vi "FYP_VI_MIDI_Virtual_Piano.vi"() -> ()   [LabVIEW 2013]
doc: "Virtual piano with LabView \nVirtual piano Demo\nMIDI\n\nUse at your own Risk"
uses:
  <vilib>/Utility/file.llb/Write To Spreadsheet File (string).vi
panel:
  in  "Exit":bool
  in  "Export File":bool
  in  "Time":u32
  in  "Table":string[][](table)
  in  "Instrument":i32(listbox)
  in  "Velocity / Volume":u32=127 max=127
  in  "MIDI Channel":u32=1 min=1 max=16
  in  "deviceID":u32
  out "MIDI Note Number":i16
  out "ScanCode":i16
  out ";":bool
  out "L":bool
  out "J":bool
  out "H":bool
  out "G":bool
  out "D":bool
  out "RShift":bool
  out "/":bool
  out ".":bool
  out ",":bool
  out "M":bool
  out "N":bool
  out "B":bool
  out "V":bool
  out "C":bool
  out "Back/S":bool
  out "X":bool
  out "-/CAP":bool
  out "0":bool
  out "9":bool
  out "7":bool
  out "6":bool
  out "4":bool
  out "3":bool
  out "2":bool
  out "]/Z":bool
  out "[/Shift":bool
  out "P":bool
  out "O":bool
  out "I":bool
  out "U":bool
  out "Y":bool
  out "T":bool
  out "R":bool
  out "E":bool
  out "W":bool
  out "Q":bool
  out "~":bool
  out "Tab":bool
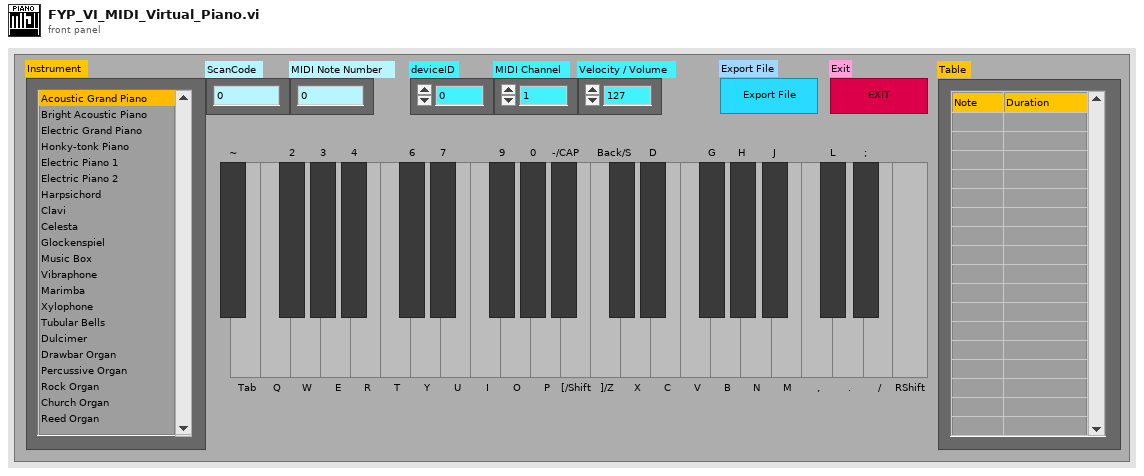
[diagram p1: front panel]
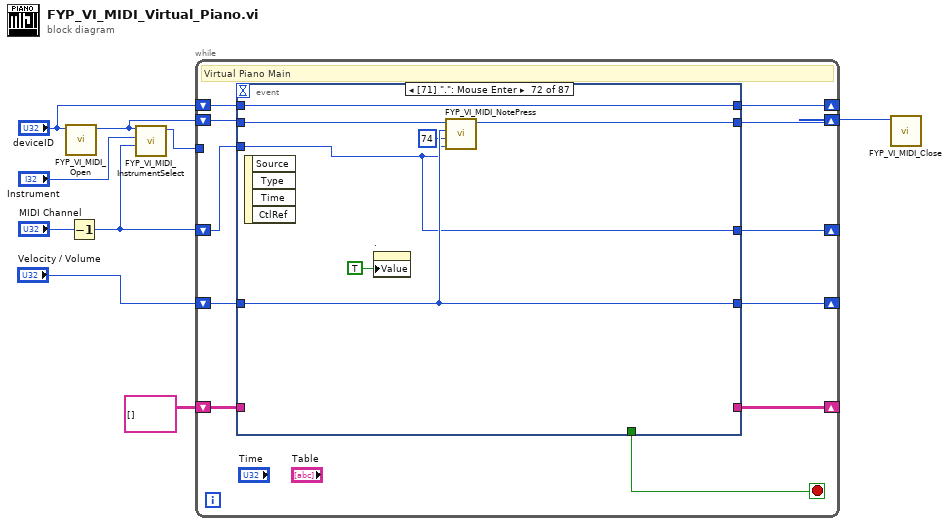
[diagram p0: block diagram]
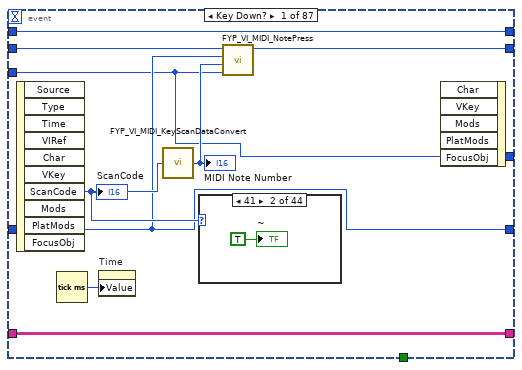
[diagram p2: hidden frame]
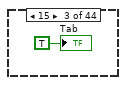
[diagram p4: hidden frame]
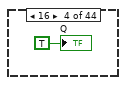
[diagram p5: hidden frame]
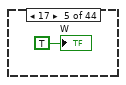
[diagram p6: hidden frame]
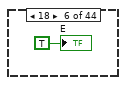
[diagram p7: hidden frame]
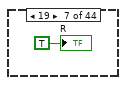
[diagram p8: hidden frame]
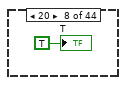
[diagram p9: hidden frame]
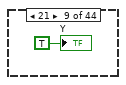
[diagram p10: hidden frame]
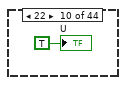
[diagram p11: hidden frame]
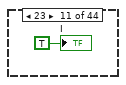
[diagram p12: hidden frame]
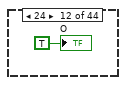
[diagram p13: hidden frame]
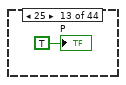
[diagram p14: hidden frame]
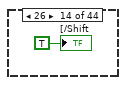
[diagram p15: hidden frame]
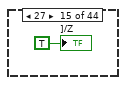
[diagram p16: hidden frame]
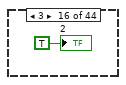
[diagram p17: hidden frame]
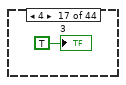
[diagram p18: hidden frame]
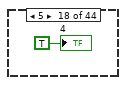
[diagram p19: hidden frame]
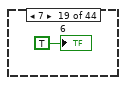
[diagram p20: hidden frame]
diagram:
  n1 = call "FYP_VI_MIDI_Open.vi"("deviceID"="deviceID") -> ("midiOut"=w5:i32)  [unwired: 5 in, 1 out]
  n2 = Decrement(x="MIDI Channel") -> (x-1=w1:u32)
  n3 = call "FYP_VI_MIDI_InstrumentSelect.vi"("MIDI Channel"=w1, "Instrument"="Instrument", "midiOut handle"=w5) -> ("midiOut handle"=w6:i32)  [unwired: 3 in, 1 out]
  n4 = while {
    shift-right: [w19] -> w8
    shift-left: w5 -> [w20]
    shift-right: [w17] -> _
    shift-left: "Velocity / Volume" -> [w18]
    tunnel: w6 -> [_]
    shift-right: [w13] -> _
    shift-left: string[][] [] ("array") -> [w14]
    shift-right: [w11] -> _
    shift-left: "deviceID" -> [w12]
    shift-right: [w10] -> _
    shift-left: w1 -> [w16]
    stop <- w15 stop-if-true
    # "Virtual Piano Main"
    n5 = event shown="[71] \".\": Mouse Enter" {
      selector: _ -> [_ _ _ _ _ _ _ _ _ _ _ _ _ _ _ _ _ _ _ _ _ _ _ _ _ _ _ _ _ _ _ _ _ _ _ _ _ _ _ _ _ _ _ _ _ _ _ _ _ _ _ _ _ _ _ _ _ _ _ _ _ _ _ _ _ _ _ _ _ _ _ _ _ _ _ _ _ _ _ _ _ _ _ _ _ _ _]
      dyn-events: _ -> [_ _ _ _ _ _ _ _ _ _ _ _ _ _ _ _ _ _ _ _ _ _ _ _ _ _ _ _ _ _ _ _ _ _ _ _ _ _ _ _ _ _ _ _ _ _ _ _ _ _ _ _ _ _ _ _ _ _ _ _ _ _ _ _ _ _ _ _ _ _ _ _ _ _ _ _ _ _ _ _ _ _ _ _ _ _ _]
      timeout: _ -> [_ _ _ _ _ _ _ _ _ _ _ _ _ _ _ _ _ _ _ _ _ _ _ _ _ _ _ _ _ _ _ _ _ _ _ _ _ _ _ _ _ _ _ _ _ _ _ _ _ _ _ _ _ _ _ _ _ _ _ _ _ _ _ _ _ _ _ _ _ _ _ _ _ _ _ _ _ _ _ _ _ _ _ _ _ _ _]
      tunnel: w20 -> [w28 w78 w85 w93 w100 w107 w114 w121 w128 w135 w142 w149 w156 w163 w170 w177 w184 w191 w198 w205 w212 w219 w226 w233 w240 w247 w254 w261 w268 w275 w282 w289 w296 w303 w309 w317 w324 w331 w338 w345 w351 w359 w366 w373 w380 w387 w393 w401 w407 w415 w422 w429 w435 w442 w450 w457 w463 w471 w478 w485 w492 w499 w505 w513 w519 w527 w533 w541 w548 w555 w562 w569 w576 w583 w590 w597 w604 w611 w618 w623 w626 w641 w687 w691 w696 w704 w705]
      tunnel: [w27 w77 w84 w92 w99 w106 w113 w120 w127 w134 w141 w148 w155 w162 w169 w176 w183 w190 w197 w204 w211 w218 w225 w232 w239 w246 w253 w260 w267 w274 w281 w288 w295 w302 w308 w316 w323 w330 w337 w344 w350 w358 w365 w372 w379 w386 w392 w400 w406 w414 w421 w428 w434 w441 w449 w456 w462 w470 w477 w484 w491 w498 w500 w512 w518 w526 w532 w540 w547 w554 w561 w563 w575 w582 w589 w596 w603 w610 w617 w623 w626 w640 w689 w691 w696 w703 w705] -> w19
      tunnel: w18 -> [w26 w76 w83 w90 w98 w105 w112 w119 w126 w133 w140 w147 w154 w161 w168 w174 w182 w189 w196 w203 w210 w217 w224 w231 w238 w245 w251 w259 w266 w273 w280 w287 w294 w301 w307 w315 w322 w329 w336 w342 w349 w357 w364 w371 w378 w385 w391 w399 w405 w413 w420 w427 w433 w440 w448 w455 w461 w469 w475 w483 w490 w497 w504 w510 w517 w525 w531 w539 w546 w553 w560 w568 w574 w581 w588 w595 w602 w609 w616 w622 w627 w639 w688 _ w698 w700 w708]
      tunnel: [w26 w76 w83 w90 w98 w105 w112 w119 w126 w133 w140 w147 w154 w161 w168 w174 w182 w189 w196 w203 w210 w217 w224 w231 w238 w245 w251 w259 w266 w273 w280 w287 w294 w301 w307 w315 w322 w329 w336 w342 w349 w357 w364 w371 w378 w385 w391 w399 w405 w413 w420 w427 w433 w440 w448 w455 w461 w469 w475 w483 w490 w497 w504 w510 w517 w525 w531 w539 w546 w553 w560 w568 w574 w581 w588 w595 w602 w609 w616 w622 w627 w639 w688 w694 w698 w700 w708] -> w17
      tunnel: w16 -> [w21 w74 w81 w87 w95 w101 w108 w115 w122 w129 w136 w143 w150 w157 w164 w171 w178 w186 w192 w200 w206 w213 w220 w227 w234 w241 w248 w255 w262 w269 w276 w283 w290 w297 w305 w312 w319 w326 w332 w339 w346 w353 w361 w367 w374 w381 w388 w395 w402 w409 w416 w423 w430 w437 w444 w451 w458 w465 w472 w480 w487 w493 w501 w507 w514 w521 w528 w535 w542 w549 w556 w564 w570 w577 w584 w591 w599 w605 w612 w621 w625 w629 w686 w693 _ w701 w707]
      tunnel: [_ _ _ _ _ _ _ _ _ _ _ _ _ _ _ _ _ _ _ _ _ _ _ _ _ _ _ _ _ _ _ _ _ _ _ _ _ _ _ _ _ _ _ _ _ _ _ _ _ _ _ _ _ _ _ _ _ _ _ _ _ _ _ _ _ _ _ _ _ _ _ _ _ _ _ _ _ _ _ "Exit" _ _ _ _ _ _ _] -> w15
      tunnel: w14 -> [w23 _ _ _ _ _ _ _ _ _ _ _ _ _ _ _ _ _ _ _ _ _ _ _ _ _ _ _ _ _ _ _ _ _ _ _ _ _ _ _ _ _ _ _ _ _ _ _ _ _ _ _ _ _ _ _ _ _ _ _ _ _ _ _ _ _ _ _ _ _ _ _ _ _ _ _ _ _ _ _ _ w634 _ _ _ _ w713]
      tunnel: [w23 _ _ _ _ _ _ _ _ _ _ _ _ _ _ _ _ _ _ _ _ _ _ _ _ _ _ _ _ _ _ _ _ _ _ _ _ _ _ _ _ _ _ _ _ _ _ _ _ _ _ _ _ _ _ _ _ _ _ _ _ _ _ _ _ _ _ _ _ _ _ _ _ _ _ _ _ _ _ _ _ w631 _ _ _ _ _] -> w13
      tunnel: w12 -> [w22 w73 w80 w88 w94 w102 w109 w116 w123 w130 w137 w144 w151 w158 w165 w172 w179 w185 w193 w199 w207 w214 w221 w228 w235 w242 w249 w256 w263 w270 w277 w284 w291 w298 w304 w311 w318 w325 w333 w340 w347 w354 w360 w368 w375 w382 w389 w396 w403 w410 w417 w424 w431 w438 w445 w452 w459 w466 w473 w479 w486 w494 w502 w508 w515 w522 w529 w536 w543 w550 w557 w565 w571 w578 w585 w592 w598 w606 w613 w620 w624 w630 w685 w692 w697 w702 w706]
      tunnel: [w22 w73 w80 w88 w94 w102 w109 w116 w123 w130 w137 w144 w151 w158 w165 w172 w179 w185 w193 w199 w207 w214 w221 w228 w235 w242 w249 w256 w263 w270 w277 w284 w291 w298 w304 w311 w318 w325 w333 w340 w347 w354 w360 w368 w375 w382 w389 w396 w403 w410 w417 w424 w431 w438 w445 w452 w459 w466 w473 w479 w486 w494 w502 w508 w515 w522 w529 w536 w543 w550 w557 w565 w571 w578 w585 w592 w598 w606 w613 w620 w624 w630 w685 w692 w697 w702 w706] -> w11
      tunnel: [w21 w74 w81 w87 w95 w101 w108 w115 w122 w129 w136 w143 w150 w157 w164 w171 w178 w186 w192 w200 w206 w213 w220 w227 w234 w241 w248 w255 w262 w269 w276 w283 w290 w297 w305 w312 w319 w326 w332 w339 w346 w353 w361 w367 w374 w381 w388 w395 w402 w409 w416 w423 w430 w437 w444 w451 w458 w465 w472 w480 w487 w493 w501 w507 w514 w521 w528 w535 w542 w549 w556 w564 w570 w577 w584 w591 w599 w605 w612 w621 w625 w629 w686 w693 w695 w701 w707] -> w10
      event Key Down? {
        n6 = event-data() -> ("ScanCode"=w29:i16)  [unwired: 1 in, 9 out]
        "ScanCode" <- w29
        n7 = Tick Count (ms)() -> (millisecond timer value=w24:u32)
        n8 = property on="Time" class="DigNum (strict)"("Value"=w24) -> ()  [unwired: 2 in, 2 out]
        n9 = call "FYP_VI_MIDI_KeyScanDataConvert.vi"("KeyScan"=w29) -> ("MIDI Note Number"=w25:i16)
        "MIDI Note Number" <- w25
        n10 = case shown="41" w29 {
          frame 0, Default {
          }
          frame 41 {
            "~" <- TRUE ("Q")
          }
          frame 15 {
            "Tab" <- TRUE ("Q")
          }
          frame 16 {
            "Q" <- TRUE ("Q")
          }
          frame 17 {
            "W" <- TRUE ("4")
          }
          frame 18 {
            "E" <- TRUE ("4")
          }
          frame 19 {
            "R" <- TRUE ("4")
          }
          frame 20 {
            "T" <- TRUE ("4")
          }
          frame 21 {
            "Y" <- TRUE ("4")
          }
          frame 22 {
            "U" <- TRUE ("4")
          }
          frame 23 {
            "I" <- TRUE ("4")
          }
          frame 24 {
            "O" <- TRUE ("4")
          }
          frame 25 {
            "P" <- TRUE ("4")
          }
          frame 26 {
            "[/Shift" <- TRUE ("4")
          }
          frame 27 {
            "]/Z" <- TRUE ("4")
          }
          frame 3 {
            "2" <- TRUE ("Q")
          }
          frame 4 {
            "3" <- TRUE ("4")
          }
          frame 5 {
            "4" <- TRUE ("4")
          }
          frame 7 {
            "6" <- TRUE ("4")
          }
          frame 8 {
            "7" <- TRUE ("4")
          }
          frame 10 {
            "9" <- TRUE ("4")
          }
          frame 11 {
            "0" <- TRUE ("4")
          }
          frame 12 {
            "-/CAP" <- TRUE ("4")
          }
          frame 14 {
            "Back/S" <- TRUE ("4")
          }
          frame 58 {
            n11 = property on="-/CAP" class="Bool"("Value"=TRUE ("4")) -> ()  [unwired: 2 in, 2 out]
          }
          frame 42 {
            n12 = local write "[/Shift"(TRUE ("4")) -> ()
          }
          frame 44 {
            n13 = local write "]/Z"(TRUE ("4")) -> ()
          }
          frame 45 {
            "X" <- TRUE ("4")
          }
          frame 46 {
            "C" <- TRUE ("4")
          }
          frame 47 {
            "V" <- TRUE ("4")
          }
          frame 48 {
            "B" <- TRUE ("4")
          }
          frame 49 {
            "N" <- TRUE ("4")
          }
          frame 50 {
            "M" <- TRUE ("4")
          }
          frame 51 {
            "," <- TRUE ("4")
          }
          frame 52 {
            "." <- TRUE ("4")
          }
          frame 53 {
            "/" <- TRUE ("4")
          }
          frame 54 {
            "RShift" <- TRUE ("4")
          }
          frame 31 {
            n14 = local write "Back/S"(TRUE ("4")) -> ()
          }
          frame 32 {
            "D" <- TRUE ("4")
          }
          frame 34 {
            "G" <- TRUE ("4")
          }
          frame 35 {
            "H" <- TRUE ("4")
          }
          frame 36 {
            "J" <- TRUE ("4")
          }
          frame 38 {
            "L" <- TRUE ("4")
          }
          frame 39 {
            ";" <- TRUE ("4")
          }
        }
        n15 = call "FYP_VI_MIDI_NotePress.vi"("MIDI Channel"=w21, "Pitch Note"=w25, "Velocity / Volume"=w26, "midiOut Handle"=w28) -> ("midiOut handle"=w27:i32)  [unwired: 2 in, 1 out]
        n16 = event-data() -> ()  [unwired: 6 in, 1 out]
      }
      event "~": Mouse Enter {
        n17 = event-data() -> ()  [unwired: 1 in, 4 out]
        n18 = property on="~" class="Bool"("Value"=TRUE ("Q")) -> ()  [unwired: 2 in, 2 out]
        n19 = call "FYP_VI_MIDI_NotePress.vi"("MIDI Channel"=w74, "Pitch Note"=u32 39, "Velocity / Volume"=w76, "midiOut Handle"=w78) -> ("midiOut handle"=w77:i32)  [unwired: 2 in, 1 out]
      }
      event "~": Mouse Leave {
        n20 = event-data() -> ()  [unwired: 1 in, 4 out]
        n21 = property on="~" class="Bool"("Value"=FALSE ("Q")) -> ()  [unwired: 2 in, 2 out]
        n22 = call "FYP_VI_MIDI_NoteRelease.vi"("MIDI Channel"=w81, "Pitch Note"=u32 39, "Velocity / Volume"=w83, "midiOut Handle"=w85) -> ("midiOut handle"=w84:i32)  [unwired: 2 in, 1 out]
      }
      event "Tab": Mouse Enter {
        n23 = event-data() -> ()  [unwired: 1 in, 4 out]
        n24 = property on="Tab" class="Bool"("Value"=TRUE ("Q")) -> ()  [unwired: 2 in, 2 out]
        n25 = call "FYP_VI_MIDI_NotePress.vi"("MIDI Channel"=w87, "Pitch Note"=u32 40, "Velocity / Volume"=w90, "midiOut Handle"=w93) -> ("midiOut handle"=w92:i32)  [unwired: 2 in, 1 out]
      }
      event "Tab": Mouse Leave {
        n26 = event-data() -> ()  [unwired: 1 in, 4 out]
        n27 = property on="Tab" class="Bool"("Value"=FALSE ("Q")) -> ()  [unwired: 2 in, 2 out]
        n28 = call "FYP_VI_MIDI_NoteRelease.vi"("MIDI Channel"=w95, "Pitch Note"=u32 40, "Velocity / Volume"=w98, "midiOut Handle"=w100) -> ("midiOut handle"=w99:i32)  [unwired: 2 in, 1 out]
      }
      event "Q": Mouse Enter {
        n29 = event-data() -> ()  [unwired: 1 in, 4 out]
        n30 = property on="Q" class="Bool"("Value"=TRUE ("Q")) -> ()  [unwired: 2 in, 2 out]
        n31 = call "FYP_VI_MIDI_NotePress.vi"("MIDI Channel"=w101, "Pitch Note"=u32 41, "Velocity / Volume"=w105, "midiOut Handle"=w107) -> ("midiOut handle"=w106:i32)  [unwired: 2 in, 1 out]
      }
      event "Q": Mouse Leave {
        n32 = event-data() -> ()  [unwired: 1 in, 4 out]
        n33 = property on="Q" class="Bool"("Value"=FALSE ("Q")) -> ()  [unwired: 2 in, 2 out]
        n34 = call "FYP_VI_MIDI_NoteRelease.vi"("MIDI Channel"=w108, "Pitch Note"=u32 41, "Velocity / Volume"=w112, "midiOut Handle"=w114) -> ("midiOut handle"=w113:i32)  [unwired: 2 in, 1 out]
      }
      event "2": Mouse Enter {
        n35 = event-data() -> ()  [unwired: 1 in, 4 out]
        n36 = property on="2" class="Bool"("Value"=TRUE ("Q")) -> ()  [unwired: 2 in, 2 out]
        n37 = call "FYP_VI_MIDI_NotePress.vi"("MIDI Channel"=w115, "Pitch Note"=u32 42, "Velocity / Volume"=w119, "midiOut Handle"=w121) -> ("midiOut handle"=w120:i32)  [unwired: 2 in, 1 out]
      }
      event "2": Mouse Leave {
        n38 = event-data() -> ()  [unwired: 1 in, 4 out]
        n39 = property on="2" class="Bool"("Value"=FALSE ("Q")) -> ()  [unwired: 2 in, 2 out]
        n40 = call "FYP_VI_MIDI_NoteRelease.vi"("MIDI Channel"=w122, "Pitch Note"=u32 42, "Velocity / Volume"=w126, "midiOut Handle"=w128) -> ("midiOut handle"=w127:i32)  [unwired: 2 in, 1 out]
      }
      event "W": Mouse Enter {
        n41 = event-data() -> ()  [unwired: 1 in, 4 out]
        n42 = property on="W" class="Bool"("Value"=TRUE ("Q")) -> ()  [unwired: 2 in, 2 out]
        n43 = call "FYP_VI_MIDI_NotePress.vi"("MIDI Channel"=w129, "Pitch Note"=u32 43, "Velocity / Volume"=w133, "midiOut Handle"=w135) -> ("midiOut handle"=w134:i32)  [unwired: 2 in, 1 out]
      }
      event "W": Mouse Leave {
        n44 = event-data() -> ()  [unwired: 1 in, 4 out]
        n45 = property on="W" class="Bool"("Value"=FALSE ("Q")) -> ()  [unwired: 2 in, 2 out]
        n46 = call "FYP_VI_MIDI_NoteRelease.vi"("MIDI Channel"=w136, "Pitch Note"=u32 43, "Velocity / Volume"=w140, "midiOut Handle"=w142) -> ("midiOut handle"=w141:i32)  [unwired: 2 in, 1 out]
      }
      event "3": Mouse Enter {
        n47 = event-data() -> ()  [unwired: 1 in, 4 out]
        n48 = property on="3" class="Bool"("Value"=TRUE ("Q")) -> ()  [unwired: 2 in, 2 out]
        n49 = call "FYP_VI_MIDI_NotePress.vi"("MIDI Channel"=w143, "Pitch Note"=u32 44, "Velocity / Volume"=w147, "midiOut Handle"=w149) -> ("midiOut handle"=w148:i32)  [unwired: 2 in, 1 out]
      }
      event "3": Mouse Leave {
        n50 = event-data() -> ()  [unwired: 1 in, 4 out]
        n51 = property on="3" class="Bool"("Value"=FALSE ("Q")) -> ()  [unwired: 2 in, 2 out]
        n52 = call "FYP_VI_MIDI_NoteRelease.vi"("MIDI Channel"=w150, "Pitch Note"=u32 44, "Velocity / Volume"=w154, "midiOut Handle"=w156) -> ("midiOut handle"=w155:i32)  [unwired: 2 in, 1 out]
      }
      event "E": Mouse Enter {
        n53 = event-data() -> ()  [unwired: 1 in, 4 out]
        n54 = property on="E" class="Bool"("Value"=TRUE ("Q")) -> ()  [unwired: 2 in, 2 out]
        n55 = call "FYP_VI_MIDI_NotePress.vi"("MIDI Channel"=w157, "Pitch Note"=u32 45, "Velocity / Volume"=w161, "midiOut Handle"=w163) -> ("midiOut handle"=w162:i32)  [unwired: 2 in, 1 out]
      }
      event "E": Mouse Leave {
        n56 = event-data() -> ()  [unwired: 1 in, 4 out]
        n57 = property on="E" class="Bool"("Value"=FALSE ("Q")) -> ()  [unwired: 2 in, 2 out]
        n58 = call "FYP_VI_MIDI_NoteRelease.vi"("MIDI Channel"=w164, "Pitch Note"=u32 45, "Velocity / Volume"=w168, "midiOut Handle"=w170) -> ("midiOut handle"=w169:i32)  [unwired: 2 in, 1 out]
      }
      event "4": Mouse Enter {
        n59 = event-data() -> ()  [unwired: 1 in, 4 out]
        n60 = property on="4" class="Bool"("Value"=TRUE ("Q")) -> ()  [unwired: 2 in, 2 out]
        n61 = call "FYP_VI_MIDI_NotePress.vi"("MIDI Channel"=w171, "Pitch Note"=u32 46, "Velocity / Volume"=w174, "midiOut Handle"=w177) -> ("midiOut handle"=w176:i32)  [unwired: 2 in, 1 out]
      }
      event "4": Mouse Leave {
        n62 = event-data() -> ()  [unwired: 1 in, 4 out]
        n63 = property on="4" class="Bool"("Value"=FALSE ("Q")) -> ()  [unwired: 2 in, 2 out]
        n64 = call "FYP_VI_MIDI_NoteRelease.vi"("MIDI Channel"=w178, "Pitch Note"=u32 46, "Velocity / Volume"=w182, "midiOut Handle"=w184) -> ("midiOut handle"=w183:i32)  [unwired: 2 in, 1 out]
      }
      event "R": Mouse Enter {
        n65 = event-data() -> ()  [unwired: 1 in, 4 out]
        n66 = property on="R" class="Bool"("Value"=TRUE ("Q")) -> ()  [unwired: 2 in, 2 out]
        n67 = call "FYP_VI_MIDI_NotePress.vi"("MIDI Channel"=w186, "Pitch Note"=u32 47, "Velocity / Volume"=w189, "midiOut Handle"=w191) -> ("midiOut handle"=w190:i32)  [unwired: 2 in, 1 out]
      }
      event "R": Mouse Leave {
        n68 = event-data() -> ()  [unwired: 1 in, 4 out]
        n69 = property on="R" class="Bool"("Value"=FALSE ("Q")) -> ()  [unwired: 2 in, 2 out]
        n70 = call "FYP_VI_MIDI_NoteRelease.vi"("MIDI Channel"=w192, "Pitch Note"=u32 47, "Velocity / Volume"=w196, "midiOut Handle"=w198) -> ("midiOut handle"=w197:i32)  [unwired: 2 in, 1 out]
      }
      event "T": Mouse Enter {
        n71 = event-data() -> ()  [unwired: 1 in, 4 out]
        n72 = property on="T" class="Bool"("Value"=TRUE ("Q")) -> ()  [unwired: 2 in, 2 out]
        n73 = call "FYP_VI_MIDI_NotePress.vi"("MIDI Channel"=w200, "Pitch Note"=u32 48, "Velocity / Volume"=w203, "midiOut Handle"=w205) -> ("midiOut handle"=w204:i32)  [unwired: 2 in, 1 out]
      }
      event "T": Mouse Leave {
        n74 = event-data() -> ()  [unwired: 1 in, 4 out]
        n75 = property on="T" class="Bool"("Value"=FALSE ("Q")) -> ()  [unwired: 2 in, 2 out]
        n76 = call "FYP_VI_MIDI_NoteRelease.vi"("MIDI Channel"=w206, "Pitch Note"=u32 48, "Velocity / Volume"=w210, "midiOut Handle"=w212) -> ("midiOut handle"=w211:i32)  [unwired: 2 in, 1 out]
      }
      event "6": Mouse Enter {
        n77 = event-data() -> ()  [unwired: 1 in, 4 out]
        n78 = property on="6" class="Bool"("Value"=TRUE ("Q")) -> ()  [unwired: 2 in, 2 out]
        n79 = call "FYP_VI_MIDI_NotePress.vi"("MIDI Channel"=w213, "Pitch Note"=u32 49, "Velocity / Volume"=w217, "midiOut Handle"=w219) -> ("midiOut handle"=w218:i32)  [unwired: 2 in, 1 out]
      }
      event "6": Mouse Leave {
        n80 = event-data() -> ()  [unwired: 1 in, 4 out]
        n81 = property on="6" class="Bool"("Value"=FALSE ("Q")) -> ()  [unwired: 2 in, 2 out]
        n82 = call "FYP_VI_MIDI_NoteRelease.vi"("MIDI Channel"=w220, "Pitch Note"=u32 49, "Velocity / Volume"=w224, "midiOut Handle"=w226) -> ("midiOut handle"=w225:i32)  [unwired: 2 in, 1 out]
      }
      event "Y": Mouse Enter {
        n83 = event-data() -> ()  [unwired: 1 in, 4 out]
        n84 = property on="Y" class="Bool"("Value"=TRUE ("Q")) -> ()  [unwired: 2 in, 2 out]
        n85 = call "FYP_VI_MIDI_NotePress.vi"("MIDI Channel"=w227, "Pitch Note"=u32 50, "Velocity / Volume"=w231, "midiOut Handle"=w233) -> ("midiOut handle"=w232:i32)  [unwired: 2 in, 1 out]
      }
      event "Y": Mouse Leave {
        n86 = event-data() -> ()  [unwired: 1 in, 4 out]
        n87 = property on="Y" class="Bool"("Value"=FALSE ("Q")) -> ()  [unwired: 2 in, 2 out]
        n88 = call "FYP_VI_MIDI_NoteRelease.vi"("MIDI Channel"=w234, "Pitch Note"=u32 50, "Velocity / Volume"=w238, "midiOut Handle"=w240) -> ("midiOut handle"=w239:i32)  [unwired: 2 in, 1 out]
      }
      event "7": Mouse Enter {
        n89 = event-data() -> ()  [unwired: 1 in, 4 out]
        n90 = property on="7" class="Bool"("Value"=TRUE ("Q")) -> ()  [unwired: 2 in, 2 out]
        n91 = call "FYP_VI_MIDI_NotePress.vi"("MIDI Channel"=w241, "Pitch Note"=u32 51, "Velocity / Volume"=w245, "midiOut Handle"=w247) -> ("midiOut handle"=w246:i32)  [unwired: 2 in, 1 out]
      }
      event "7": Mouse Leave {
        n92 = event-data() -> ()  [unwired: 1 in, 4 out]
        n93 = property on="7" class="Bool"("Value"=FALSE ("Q")) -> ()  [unwired: 2 in, 2 out]
        n94 = call "FYP_VI_MIDI_NoteRelease.vi"("MIDI Channel"=w248, "Pitch Note"=u32 51, "Velocity / Volume"=w251, "midiOut Handle"=w254) -> ("midiOut handle"=w253:i32)  [unwired: 2 in, 1 out]
      }
      event "U": Mouse Enter {
        n95 = event-data() -> ()  [unwired: 1 in, 4 out]
        n96 = property on="U" class="Bool"("Value"=TRUE ("Q")) -> ()  [unwired: 2 in, 2 out]
        n97 = call "FYP_VI_MIDI_NotePress.vi"("MIDI Channel"=w255, "Pitch Note"=u32 52, "Velocity / Volume"=w259, "midiOut Handle"=w261) -> ("midiOut handle"=w260:i32)  [unwired: 2 in, 1 out]
      }
      event "U": Mouse Leave {
        n98 = event-data() -> ()  [unwired: 1 in, 4 out]
        n99 = property on="U" class="Bool"("Value"=FALSE ("Q")) -> ()  [unwired: 2 in, 2 out]
        n100 = call "FYP_VI_MIDI_NoteRelease.vi"("MIDI Channel"=w262, "Pitch Note"=u32 52, "Velocity / Volume"=w266, "midiOut Handle"=w268) -> ("midiOut handle"=w267:i32)  [unwired: 2 in, 1 out]
      }
      event "I": Mouse Enter {
        n101 = event-data() -> ()  [unwired: 1 in, 4 out]
        n102 = property on="I" class="Bool"("Value"=TRUE ("Q")) -> ()  [unwired: 2 in, 2 out]
        n103 = call "FYP_VI_MIDI_NotePress.vi"("MIDI Channel"=w269, "Pitch Note"=u32 53, "Velocity / Volume"=w273, "midiOut Handle"=w275) -> ("midiOut handle"=w274:i32)  [unwired: 2 in, 1 out]
      }
      event "I": Mouse Leave {
        n104 = event-data() -> ()  [unwired: 1 in, 4 out]
        n105 = property on="I" class="Bool"("Value"=FALSE ("Q")) -> ()  [unwired: 2 in, 2 out]
        n106 = call "FYP_VI_MIDI_NoteRelease.vi"("MIDI Channel"=w276, "Pitch Note"=u32 53, "Velocity / Volume"=w280, "midiOut Handle"=w282) -> ("midiOut handle"=w281:i32)  [unwired: 2 in, 1 out]
      }
      event "9": Mouse Enter {
        n107 = event-data() -> ()  [unwired: 1 in, 4 out]
        n108 = property on="9" class="Bool"("Value"=TRUE ("Q")) -> ()  [unwired: 2 in, 2 out]
        n109 = call "FYP_VI_MIDI_NotePress.vi"("MIDI Channel"=w283, "Pitch Note"=u32 54, "Velocity / Volume"=w287, "midiOut Handle"=w289) -> ("midiOut handle"=w288:i32)  [unwired: 2 in, 1 out]
      }
      event "9": Mouse Leave {
        n110 = event-data() -> ()  [unwired: 1 in, 4 out]
        n111 = property on="9" class="Bool"("Value"=FALSE ("Q")) -> ()  [unwired: 2 in, 2 out]
        n112 = call "FYP_VI_MIDI_NoteRelease.vi"("MIDI Channel"=w290, "Pitch Note"=u32 54, "Velocity / Volume"=w294, "midiOut Handle"=w296) -> ("midiOut handle"=w295:i32)  [unwired: 2 in, 1 out]
      }
      event "O": Mouse Enter {
        n113 = event-data() -> ()  [unwired: 1 in, 4 out]
        n114 = property on="O" class="Bool"("Value"=TRUE ("Q")) -> ()  [unwired: 2 in, 2 out]
        n115 = call "FYP_VI_MIDI_NotePress.vi"("MIDI Channel"=w297, "Pitch Note"=u32 55, "Velocity / Volume"=w301, "midiOut Handle"=w303) -> ("midiOut handle"=w302:i32)  [unwired: 2 in, 1 out]
      }
      event "O": Mouse Leave {
        n116 = event-data() -> ()  [unwired: 1 in, 4 out]
        n117 = property on="O" class="Bool"("Value"=FALSE ("Q")) -> ()  [unwired: 2 in, 2 out]
        n118 = call "FYP_VI_MIDI_NoteRelease.vi"("MIDI Channel"=w305, "Pitch Note"=u32 55, "Velocity / Volume"=w307, "midiOut Handle"=w309) -> ("midiOut handle"=w308:i32)  [unwired: 2 in, 1 out]
      }
      event "0": Mouse Enter {
        n119 = event-data() -> ()  [unwired: 1 in, 4 out]
        n120 = property on="0" class="Bool"("Value"=TRUE ("Q")) -> ()  [unwired: 2 in, 2 out]
        n121 = call "FYP_VI_MIDI_NotePress.vi"("MIDI Channel"=w312, "Pitch Note"=u32 56, "Velocity / Volume"=w315, "midiOut Handle"=w317) -> ("midiOut handle"=w316:i32)  [unwired: 2 in, 1 out]
      }
      event "0": Mouse Leave {
        n122 = event-data() -> ()  [unwired: 1 in, 4 out]
        n123 = property on="0" class="Bool"("Value"=FALSE ("Q")) -> ()  [unwired: 2 in, 2 out]
        n124 = call "FYP_VI_MIDI_NoteRelease.vi"("MIDI Channel"=w319, "Pitch Note"=u32 56, "Velocity / Volume"=w322, "midiOut Handle"=w324) -> ("midiOut handle"=w323:i32)  [unwired: 2 in, 1 out]
      }
      event "P": Mouse Enter {
        n125 = event-data() -> ()  [unwired: 1 in, 4 out]
        n126 = property on="P" class="Bool"("Value"=TRUE ("Q")) -> ()  [unwired: 2 in, 2 out]
        n127 = call "FYP_VI_MIDI_NotePress.vi"("MIDI Channel"=w326, "Pitch Note"=u32 57, "Velocity / Volume"=w329, "midiOut Handle"=w331) -> ("midiOut handle"=w330:i32)  [unwired: 2 in, 1 out]
      }
      event "P": Mouse Leave {
        n128 = event-data() -> ()  [unwired: 1 in, 4 out]
        n129 = property on="P" class="Bool"("Value"=FALSE ("Q")) -> ()  [unwired: 2 in, 2 out]
        n130 = call "FYP_VI_MIDI_NoteRelease.vi"("MIDI Channel"=w332, "Pitch Note"=u32 57, "Velocity / Volume"=w336, "midiOut Handle"=w338) -> ("midiOut handle"=w337:i32)  [unwired: 2 in, 1 out]
      }
      event "-/CAP": Mouse Enter {
        n131 = event-data() -> ()  [unwired: 1 in, 4 out]
        n132 = property on="-/CAP" class="Bool"("Value"=TRUE ("Q")) -> ()  [unwired: 2 in, 2 out]
        n133 = call "FYP_VI_MIDI_NotePress.vi"("MIDI Channel"=w339, "Pitch Note"=u32 58, "Velocity / Volume"=w342, "midiOut Handle"=w345) -> ("midiOut handle"=w344:i32)  [unwired: 2 in, 1 out]
      }
      event "-/CAP": Mouse Leave {
        n134 = event-data() -> ()  [unwired: 1 in, 4 out]
        n135 = property on="-/CAP" class="Bool"("Value"=FALSE ("Q")) -> ()  [unwired: 2 in, 2 out]
        n136 = call "FYP_VI_MIDI_NoteRelease.vi"("MIDI Channel"=w346, "Pitch Note"=u32 58, "Velocity / Volume"=w349, "midiOut Handle"=w351) -> ("midiOut handle"=w350:i32)  [unwired: 2 in, 1 out]
      }
      event "[/Shift": Mouse Enter {
        n137 = event-data() -> ()  [unwired: 1 in, 4 out]
        n138 = property on="[/Shift" class="Bool"("Value"=TRUE ("Q")) -> ()  [unwired: 2 in, 2 out]
        n139 = call "FYP_VI_MIDI_NotePress.vi"("MIDI Channel"=w353, "Pitch Note"=u32 59, "Velocity / Volume"=w357, "midiOut Handle"=w359) -> ("midiOut handle"=w358:i32)  [unwired: 2 in, 1 out]
      }
      event "[/Shift": Mouse Leave {
        n140 = event-data() -> ()  [unwired: 1 in, 4 out]
        n141 = property on="[/Shift" class="Bool"("Value"=FALSE ("Q")) -> ()  [unwired: 2 in, 2 out]
        n142 = call "FYP_VI_MIDI_NoteRelease.vi"("MIDI Channel"=w361, "Pitch Note"=u32 59, "Velocity / Volume"=w364, "midiOut Handle"=w366) -> ("midiOut handle"=w365:i32)  [unwired: 2 in, 1 out]
      }
      event "]/Z": Mouse Enter {
        n143 = event-data() -> ()  [unwired: 1 in, 4 out]
        n144 = property on="]/Z" class="Bool"("Value"=TRUE ("Q")) -> ()  [unwired: 2 in, 2 out]
        n145 = call "FYP_VI_MIDI_NotePress.vi"("MIDI Channel"=w367, "Pitch Note"=u32 60, "Velocity / Volume"=w371, "midiOut Handle"=w373) -> ("midiOut handle"=w372:i32)  [unwired: 2 in, 1 out]
      }
      event "]/Z": Mouse Leave {
        n146 = event-data() -> ()  [unwired: 1 in, 4 out]
        n147 = property on="]/Z" class="Bool"("Value"=FALSE ("Q")) -> ()  [unwired: 2 in, 2 out]
        n148 = call "FYP_VI_MIDI_NoteRelease.vi"("MIDI Channel"=w374, "Pitch Note"=u32 60, "Velocity / Volume"=w378, "midiOut Handle"=w380) -> ("midiOut handle"=w379:i32)  [unwired: 2 in, 1 out]
      }
      event "Back/S": Mouse Enter {
        n149 = event-data() -> ()  [unwired: 1 in, 4 out]
        n150 = property on="Back/S" class="Bool"("Value"=TRUE ("Q")) -> ()  [unwired: 2 in, 2 out]
        n151 = call "FYP_VI_MIDI_NotePress.vi"("MIDI Channel"=w381, "Pitch Note"=u32 61, "Velocity / Volume"=w385, "midiOut Handle"=w387) -> ("midiOut handle"=w386:i32)  [unwired: 2 in, 1 out]
      }
      event "Back/S": Mouse Leave {
        n152 = event-data() -> ()  [unwired: 1 in, 4 out]
        n153 = property on="Back/S" class="Bool"("Value"=FALSE ("Q")) -> ()  [unwired: 2 in, 2 out]
        n154 = call "FYP_VI_MIDI_NoteRelease.vi"("MIDI Channel"=w388, "Pitch Note"=u32 61, "Velocity / Volume"=w391, "midiOut Handle"=w393) -> ("midiOut handle"=w392:i32)  [unwired: 2 in, 1 out]
      }
      event "X": Mouse Enter {
        n155 = event-data() -> ()  [unwired: 1 in, 4 out]
        n156 = property on="X" class="Bool"("Value"=TRUE ("Q")) -> ()  [unwired: 2 in, 2 out]
        n157 = call "FYP_VI_MIDI_NotePress.vi"("MIDI Channel"=w395, "Pitch Note"=u32 62, "Velocity / Volume"=w399, "midiOut Handle"=w401) -> ("midiOut handle"=w400:i32)  [unwired: 2 in, 1 out]
      }
      event "X": Mouse Leave {
        n158 = event-data() -> ()  [unwired: 1 in, 4 out]
        n159 = property on="X" class="Bool"("Value"=FALSE ("Q")) -> ()  [unwired: 2 in, 2 out]
        n160 = call "FYP_VI_MIDI_NoteRelease.vi"("MIDI Channel"=w402, "Pitch Note"=u32 62, "Velocity / Volume"=w405, "midiOut Handle"=w407) -> ("midiOut handle"=w406:i32)  [unwired: 2 in, 1 out]
      }
      event "D": Mouse Enter {
        n161 = event-data() -> ()  [unwired: 1 in, 4 out]
        n162 = property on="D" class="Bool"("Value"=TRUE ("Q")) -> ()  [unwired: 2 in, 2 out]
        n163 = call "FYP_VI_MIDI_NotePress.vi"("MIDI Channel"=w409, "Pitch Note"=u32 63, "Velocity / Volume"=w413, "midiOut Handle"=w415) -> ("midiOut handle"=w414:i32)  [unwired: 2 in, 1 out]
      }
      event "D": Mouse Leave {
        n164 = event-data() -> ()  [unwired: 1 in, 4 out]
        n165 = property on="D" class="Bool"("Value"=FALSE ("Q")) -> ()  [unwired: 2 in, 2 out]
        n166 = call "FYP_VI_MIDI_NoteRelease.vi"("MIDI Channel"=w416, "Pitch Note"=u32 63, "Velocity / Volume"=w420, "midiOut Handle"=w422) -> ("midiOut handle"=w421:i32)  [unwired: 2 in, 1 out]
      }
      event "C": Mouse Enter {
        n167 = event-data() -> ()  [unwired: 1 in, 4 out]
        n168 = property on="C" class="Bool"("Value"=TRUE ("Q")) -> ()  [unwired: 2 in, 2 out]
        n169 = call "FYP_VI_MIDI_NotePress.vi"("MIDI Channel"=w423, "Pitch Note"=u32 64, "Velocity / Volume"=w427, "midiOut Handle"=w429) -> ("midiOut handle"=w428:i32)  [unwired: 2 in, 1 out]
      }
      event "C": Mouse Leave {
        n170 = event-data() -> ()  [unwired: 1 in, 4 out]
        n171 = property on="C" class="Bool"("Value"=FALSE ("Q")) -> ()  [unwired: 2 in, 2 out]
        n172 = call "FYP_VI_MIDI_NoteRelease.vi"("MIDI Channel"=w430, "Pitch Note"=u32 64, "Velocity / Volume"=w433, "midiOut Handle"=w435) -> ("midiOut handle"=w434:i32)  [unwired: 2 in, 1 out]
      }
      event "V": Mouse Enter {
        n173 = event-data() -> ()  [unwired: 1 in, 4 out]
        n174 = property on="V" class="Bool"("Value"=TRUE ("Q")) -> ()  [unwired: 2 in, 2 out]
        n175 = call "FYP_VI_MIDI_NotePress.vi"("MIDI Channel"=w437, "Pitch Note"=u32 65, "Velocity / Volume"=w440, "midiOut Handle"=w442) -> ("midiOut handle"=w441:i32)  [unwired: 2 in, 1 out]
      }
      event "V": Mouse Leave {
        n176 = event-data() -> ()  [unwired: 1 in, 4 out]
        n177 = property on="V" class="Bool"("Value"=FALSE ("Q")) -> ()  [unwired: 2 in, 2 out]
        n178 = call "FYP_VI_MIDI_NoteRelease.vi"("MIDI Channel"=w444, "Pitch Note"=u32 65, "Velocity / Volume"=w448, "midiOut Handle"=w450) -> ("midiOut handle"=w449:i32)  [unwired: 2 in, 1 out]
      }
      event "G": Mouse Enter {
        n179 = event-data() -> ()  [unwired: 1 in, 4 out]
        n180 = property on="G" class="Bool"("Value"=TRUE ("Q")) -> ()  [unwired: 2 in, 2 out]
        n181 = call "FYP_VI_MIDI_NotePress.vi"("MIDI Channel"=w451, "Pitch Note"=u32 66, "Velocity / Volume"=w455, "midiOut Handle"=w457) -> ("midiOut handle"=w456:i32)  [unwired: 2 in, 1 out]
      }
      event "G": Mouse Leave {
        n182 = event-data() -> ()  [unwired: 1 in, 4 out]
        n183 = property on="G" class="Bool"("Value"=FALSE ("Q")) -> ()  [unwired: 2 in, 2 out]
        n184 = call "FYP_VI_MIDI_NoteRelease.vi"("MIDI Channel"=w458, "Pitch Note"=u32 66, "Velocity / Volume"=w461, "midiOut Handle"=w463) -> ("midiOut handle"=w462:i32)  [unwired: 2 in, 1 out]
      }
      event "B": Mouse Enter {
        n185 = event-data() -> ()  [unwired: 1 in, 4 out]
        n186 = property on="B" class="Bool"("Value"=TRUE ("Q")) -> ()  [unwired: 2 in, 2 out]
        n187 = call "FYP_VI_MIDI_NotePress.vi"("MIDI Channel"=w465, "Pitch Note"=u32 67, "Velocity / Volume"=w469, "midiOut Handle"=w471) -> ("midiOut handle"=w470:i32)  [unwired: 2 in, 1 out]
      }
      event "B": Mouse Leave {
        n188 = event-data() -> ()  [unwired: 1 in, 4 out]
        n189 = property on="B" class="Bool"("Value"=FALSE ("Q")) -> ()  [unwired: 2 in, 2 out]
        n190 = call "FYP_VI_MIDI_NoteRelease.vi"("MIDI Channel"=w472, "Pitch Note"=u32 67, "Velocity / Volume"=w475, "midiOut Handle"=w478) -> ("midiOut handle"=w477:i32)  [unwired: 2 in, 1 out]
      }
      event "H": Mouse Enter {
        n191 = event-data() -> ()  [unwired: 1 in, 4 out]
        n192 = property on="H" class="Bool"("Value"=TRUE ("Q")) -> ()  [unwired: 2 in, 2 out]
        n193 = call "FYP_VI_MIDI_NotePress.vi"("MIDI Channel"=w480, "Pitch Note"=u32 68, "Velocity / Volume"=w483, "midiOut Handle"=w485) -> ("midiOut handle"=w484:i32)  [unwired: 2 in, 1 out]
      }
      event "H": Mouse Leave {
        n194 = event-data() -> ()  [unwired: 1 in, 4 out]
        n195 = property on="H" class="Bool"("Value"=FALSE ("Q")) -> ()  [unwired: 2 in, 2 out]
        n196 = call "FYP_VI_MIDI_NoteRelease.vi"("MIDI Channel"=w487, "Pitch Note"=u32 68, "Velocity / Volume"=w490, "midiOut Handle"=w492) -> ("midiOut handle"=w491:i32)  [unwired: 2 in, 1 out]
      }
      event "N": Mouse Enter {
        n197 = event-data() -> ()  [unwired: 1 in, 4 out]
        n198 = property on="N" class="Bool"("Value"=TRUE ("Q")) -> ()  [unwired: 2 in, 2 out]
        n199 = call "FYP_VI_MIDI_NotePress.vi"("MIDI Channel"=w493, "Pitch Note"=u32 69, "Velocity / Volume"=w497, "midiOut Handle"=w499) -> ("midiOut handle"=w498:i32)  [unwired: 2 in, 1 out]
      }
      event "N": Mouse Leave {
        n200 = event-data() -> ()  [unwired: 1 in, 4 out]
        n201 = property on="N" class="Bool"("Value"=FALSE ("Q")) -> ()  [unwired: 2 in, 2 out]
        n202 = call "FYP_VI_MIDI_NoteRelease.vi"("MIDI Channel"=w501, "Pitch Note"=u32 69, "Velocity / Volume"=w504, "midiOut Handle"=w505) -> ("midiOut handle"=w500:i32)  [unwired: 2 in, 1 out]
      }
      event "J": Mouse Enter {
        n203 = event-data() -> ()  [unwired: 1 in, 4 out]
        n204 = property on="J" class="Bool"("Value"=TRUE ("Q")) -> ()  [unwired: 2 in, 2 out]
        n205 = call "FYP_VI_MIDI_NotePress.vi"("MIDI Channel"=w507, "Pitch Note"=u32 70, "Velocity / Volume"=w510, "midiOut Handle"=w513) -> ("midiOut handle"=w512:i32)  [unwired: 2 in, 1 out]
      }
      event "J": Mouse Leave {
        n206 = event-data() -> ()  [unwired: 1 in, 4 out]
        n207 = property on="J" class="Bool"("Value"=FALSE ("Q")) -> ()  [unwired: 2 in, 2 out]
        n208 = call "FYP_VI_MIDI_NoteRelease.vi"("MIDI Channel"=w514, "Pitch Note"=u32 70, "Velocity / Volume"=w517, "midiOut Handle"=w519) -> ("midiOut handle"=w518:i32)  [unwired: 2 in, 1 out]
      }
      event "M": Mouse Enter {
        n209 = event-data() -> ()  [unwired: 1 in, 4 out]
        n210 = property on="M" class="Bool"("Value"=TRUE ("Q")) -> ()  [unwired: 2 in, 2 out]
        n211 = call "FYP_VI_MIDI_NotePress.vi"("MIDI Channel"=w521, "Pitch Note"=u32 71, "Velocity / Volume"=w525, "midiOut Handle"=w527) -> ("midiOut handle"=w526:i32)  [unwired: 2 in, 1 out]
      }
      event "M": Mouse Leave {
        n212 = event-data() -> ()  [unwired: 1 in, 4 out]
        n213 = property on="M" class="Bool"("Value"=FALSE ("Q")) -> ()  [unwired: 2 in, 2 out]
        n214 = call "FYP_VI_MIDI_NoteRelease.vi"("MIDI Channel"=w528, "Pitch Note"=u32 71, "Velocity / Volume"=w531, "midiOut Handle"=w533) -> ("midiOut handle"=w532:i32)  [unwired: 2 in, 1 out]
      }
      event ",": Mouse Enter {
        n215 = event-data() -> ()  [unwired: 1 in, 4 out]
        n216 = property on="," class="Bool"("Value"=TRUE ("Q")) -> ()  [unwired: 2 in, 2 out]
        n217 = call "FYP_VI_MIDI_NotePress.vi"("MIDI Channel"=w535, "Pitch Note"=u32 72, "Velocity / Volume"=w539, "midiOut Handle"=w541) -> ("midiOut handle"=w540:i32)  [unwired: 2 in, 1 out]
      }
      event ",": Mouse Leave {
        n218 = event-data() -> ()  [unwired: 1 in, 4 out]
        n219 = property on="," class="Bool"("Value"=FALSE ("Q")) -> ()  [unwired: 2 in, 2 out]
        n220 = call "FYP_VI_MIDI_NoteRelease.vi"("MIDI Channel"=w542, "Pitch Note"=u32 72, "Velocity / Volume"=w546, "midiOut Handle"=w548) -> ("midiOut handle"=w547:i32)  [unwired: 2 in, 1 out]
      }
      event "L": Mouse Enter {
        n221 = event-data() -> ()  [unwired: 1 in, 4 out]
        n222 = property on="L" class="Bool"("Value"=TRUE ("Q")) -> ()  [unwired: 2 in, 2 out]
        n223 = call "FYP_VI_MIDI_NotePress.vi"("MIDI Channel"=w549, "Pitch Note"=u32 73, "Velocity / Volume"=w553, "midiOut Handle"=w555) -> ("midiOut handle"=w554:i32)  [unwired: 2 in, 1 out]
      }
      event "L": Mouse Leave {
        n224 = event-data() -> ()  [unwired: 1 in, 4 out]
        n225 = property on="L" class="Bool"("Value"=FALSE ("Q")) -> ()  [unwired: 2 in, 2 out]
        n226 = call "FYP_VI_MIDI_NoteRelease.vi"("MIDI Channel"=w556, "Pitch Note"=u32 73, "Velocity / Volume"=w560, "midiOut Handle"=w562) -> ("midiOut handle"=w561:i32)  [unwired: 2 in, 1 out]
      }
      event ".": Mouse Enter {
        n227 = event-data() -> ()  [unwired: 1 in, 4 out]
        n228 = property on="." class="Bool"("Value"=TRUE ("Q")) -> ()  [unwired: 2 in, 2 out]
        n229 = call "FYP_VI_MIDI_NotePress.vi"("MIDI Channel"=w564, "Pitch Note"=u32 74, "Velocity / Volume"=w568, "midiOut Handle"=w569) -> ("midiOut handle"=w563:i32)  [unwired: 2 in, 1 out]
      }
      event ".": Mouse Leave {
        n230 = event-data() -> ()  [unwired: 1 in, 4 out]
        n231 = property on="." class="Bool"("Value"=FALSE ("Q")) -> ()  [unwired: 2 in, 2 out]
        n232 = call "FYP_VI_MIDI_NoteRelease.vi"("MIDI Channel"=w570, "Pitch Note"=u32 74, "Velocity / Volume"=w574, "midiOut Handle"=w576) -> ("midiOut handle"=w575:i32)  [unwired: 2 in, 1 out]
      }
      event ";": Mouse Enter {
        n233 = event-data() -> ()  [unwired: 1 in, 4 out]
        n234 = property on=";" class="Bool"("Value"=TRUE ("Q")) -> ()  [unwired: 2 in, 2 out]
        n235 = call "FYP_VI_MIDI_NotePress.vi"("MIDI Channel"=w577, "Pitch Note"=u32 75, "Velocity / Volume"=w581, "midiOut Handle"=w583) -> ("midiOut handle"=w582:i32)  [unwired: 2 in, 1 out]
      }
      event ";": Mouse Leave {
        n236 = event-data() -> ()  [unwired: 1 in, 4 out]
        n237 = property on=";" class="Bool"("Value"=FALSE ("Q")) -> ()  [unwired: 2 in, 2 out]
        n238 = call "FYP_VI_MIDI_NoteRelease.vi"("MIDI Channel"=w584, "Pitch Note"=u32 75, "Velocity / Volume"=w588, "midiOut Handle"=w590) -> ("midiOut handle"=w589:i32)  [unwired: 2 in, 1 out]
      }
      event "/": Mouse Enter {
        n239 = event-data() -> ()  [unwired: 1 in, 4 out]
        n240 = property on="/" class="Bool"("Value"=TRUE ("Q")) -> ()  [unwired: 2 in, 2 out]
        n241 = call "FYP_VI_MIDI_NotePress.vi"("MIDI Channel"=w591, "Pitch Note"=u32 76, "Velocity / Volume"=w595, "midiOut Handle"=w597) -> ("midiOut handle"=w596:i32)  [unwired: 2 in, 1 out]
      }
      event "/": Mouse Leave {
        n242 = event-data() -> ()  [unwired: 1 in, 4 out]
        n243 = property on="/" class="Bool"("Value"=FALSE ("Q")) -> ()  [unwired: 2 in, 2 out]
        n244 = call "FYP_VI_MIDI_NoteRelease.vi"("MIDI Channel"=w599, "Pitch Note"=u32 76, "Velocity / Volume"=w602, "midiOut Handle"=w604) -> ("midiOut handle"=w603:i32)  [unwired: 2 in, 1 out]
      }
      event "RShift": Mouse Enter {
        n245 = event-data() -> ()  [unwired: 1 in, 4 out]
        n246 = property on="RShift" class="Bool"("Value"=TRUE ("Q")) -> ()  [unwired: 2 in, 2 out]
        n247 = call "FYP_VI_MIDI_NotePress.vi"("MIDI Channel"=w605, "Pitch Note"=u32 77, "Velocity / Volume"=w609, "midiOut Handle"=w611) -> ("midiOut handle"=w610:i32)  [unwired: 2 in, 1 out]
      }
      event "RShift": Mouse Leave {
        n248 = event-data() -> ()  [unwired: 1 in, 4 out]
        n249 = property on="RShift" class="Bool"("Value"=FALSE ("Q")) -> ()  [unwired: 2 in, 2 out]
        n250 = call "FYP_VI_MIDI_NoteRelease.vi"("MIDI Channel"=w612, "Pitch Note"=u32 77, "Velocity / Volume"=w616, "midiOut Handle"=w618) -> ("midiOut handle"=w617:i32)  [unwired: 2 in, 1 out]
      }
      event "Exit": Value Change {
        n251 = event-data() -> ()  [unwired: 1 in, 6 out]
      }
      event "Instrument": Key Down?; "Instrument": event type 3.0.x8000000b {
        n252 = event-data() -> ()  [unwired: 1 in, 8 out]
        n253 = event-data("Discard?"=TRUE) -> ()  [unwired: 6 in, 1 out]
      }
      event Key Up {
        n254 = event-data() -> ("ScanCode"=w633:i16)  [unwired: 1 in, 7 out]
        n255 = property on="Time" class="DigNum (strict)"() -> ("Value"=w635:u32)  [unwired: 2 in, 2 out]
        n256 = Tick Count (ms)() -> (millisecond timer value=w636:u32)
        n257 = Subtract(x=w636, y=w635) -> (x-y=w632:u32)
        n258 = call "FYP_VI_MIDI_KeyScanDataConvert.vi"("KeyScan"=w633) -> ("MIDI Note Number"=w637:i16)
        n259 = case shown="41" w633 {
          frame 0, Default {
          }
          frame 41 {
            n260 = local write "~"(FALSE ("Q")) -> ()
          }
          frame 15 {
            n261 = local write "Tab"(FALSE ("Q")) -> ()
          }
          frame 16 {
            n262 = local write "Q"(FALSE ("Q")) -> ()
          }
          frame 17 {
            n263 = local write "W"(FALSE ("4")) -> ()
          }
          frame 18 {
            n264 = local write "E"(FALSE ("4")) -> ()
          }
          frame 19 {
            n265 = local write "R"(FALSE ("4")) -> ()
          }
          frame 20 {
            n266 = local write "T"(FALSE ("4")) -> ()
          }
          frame 21 {
            n267 = local write "Y"(FALSE ("4")) -> ()
          }
          frame 22 {
            n268 = local write "U"(FALSE ("4")) -> ()
          }
          frame 23 {
            n269 = local write "I"(FALSE ("4")) -> ()
          }
          frame 24 {
            n270 = local write "O"(FALSE ("4")) -> ()
          }
          frame 25 {
            n271 = local write "P"(FALSE ("4")) -> ()
          }
          frame 26 {
            n272 = local write "[/Shift"(FALSE ("4")) -> ()
          }
          frame 27 {
            n273 = local write "]/Z"(FALSE ("4")) -> ()
          }
          frame 3 {
            n274 = local write "2"(FALSE ("Q")) -> ()
          }
          frame 4 {
            n275 = local write "3"(FALSE ("3")) -> ()
          }
          frame 5 {
            n276 = local write "4"(FALSE ("4")) -> ()
          }
          frame 7 {
            n277 = local write "6"(FALSE ("4")) -> ()
          }
          frame 8 {
            n278 = local write "7"(FALSE ("4")) -> ()
          }
          frame 10 {
            n279 = local write "9"(FALSE ("4")) -> ()
          }
          frame 11 {
            n280 = local write "0"(FALSE ("4")) -> ()
          }
          frame 12 {
            n281 = local write "-/CAP"(FALSE ("4")) -> ()
          }
          frame 14 {
            n282 = local write "Back/S"(FALSE ("4")) -> ()
          }
          frame 58 {
            n283 = local write "-/CAP"(FALSE ("4")) -> ()
          }
          frame 42 {
            n284 = local write "[/Shift"(FALSE ("4")) -> ()
          }
          frame 44 {
            n285 = local write "]/Z"(FALSE ("4")) -> ()
          }
          frame 45 {
            n286 = local write "X"(FALSE ("4")) -> ()
          }
          frame 46 {
            n287 = local write "C"(FALSE ("4")) -> ()
          }
          frame 47 {
            n288 = local write "V"(FALSE ("4")) -> ()
          }
          frame 48 {
            n289 = local write "B"(FALSE ("4")) -> ()
          }
          frame 49 {
            n290 = local write "N"(FALSE ("4")) -> ()
          }
          frame 50 {
            n291 = local write "M"(FALSE ("4")) -> ()
          }
          frame 51 {
            n292 = local write ","(FALSE ("4")) -> ()
          }
          frame 52 {
            n293 = local write "."(FALSE ("4")) -> ()
          }
          frame 53 {
            n294 = local write "/"(FALSE ("4")) -> ()
          }
          frame 54 {
            n295 = local write "RShift"(FALSE ("4")) -> ()
          }
          frame 31 {
            n296 = local write "Back/S"(FALSE ("4")) -> ()
          }
          frame 32 {
            n297 = local write "D"(FALSE ("4")) -> ()
          }
          frame 34 {
            n298 = local write "G"(FALSE ("4")) -> ()
          }
          frame 35 {
            n299 = local write "H"(FALSE ("4")) -> ()
          }
          frame 36 {
            n300 = local write "J"(FALSE ("4")) -> ()
          }
          frame 38 {
            n301 = local write "L"(FALSE ("4")) -> ()
          }
          frame 39 {
            n302 = local write ";"(FALSE ("4")) -> ()
          }
        }
        n303 = call "FYP_VI_MIDI_NoteRelease.vi"("MIDI Channel"=w629, "Pitch Note"=w637, "Velocity / Volume"=u32 0, "midiOut Handle"=w641) -> ("midiOut handle"=w640:i32)  [unwired: 2 in, 1 out]
        n304 = call "FYP_VI_MIDI_TableData.vi"("input 2"=w632, "input 1"=w633, "array"=w634) -> ("output array"=w631:string[][])
        n305 = property on="Table" class="Tbl (strict)"("Value"=w631) -> ()  [unwired: 2 in, 2 out]
      }
      event "Instrument": Value Change {
        n306 = event-data() -> ("NewVal"=w690:i32)  [unwired: 1 in, 5 out]
        n307 = call "FYP_VI_MIDI_InstrumentSelect.vi"("MIDI Channel"=w686, "Instrument"=w690, "midiOut handle"=w687) -> ("midiOut handle"=w689:i32)  [unwired: 3 in, 1 out]
      }
      event "Velocity / Volume": Value Change {
        n308 = event-data() -> ("NewVal"=w694:u32)  [unwired: 1 in, 5 out]
      }
      event "MIDI Channel": Value Change {
        n309 = event-data() -> ("NewVal"=w699:u32)  [unwired: 1 in, 5 out]
        n310 = Decrement(x=w699) -> (x-1=w695:u32)
      }
      event "deviceID": Value Change {
        n311 = event-data() -> ()  [unwired: 1 in, 6 out]
        n312 = call "FYP_VI_MIDI_Close.vi"("midiOut"=w704) -> ()  [unwired: 6 in, 1 out]
        n313 = call "FYP_VI_MIDI_Open.vi"("deviceID"=w702) -> ("midiOut"=w703:i32)  [unwired: 5 in, 1 out]
      }
      event "Export File": Value Change {
        # "Export Data to File, .xls , .txt and other"
        n314 = event-data() -> ()  [unwired: 1 in, 6 out]
        n315 = call-poly <vilib>:"Write To Spreadsheet File.vi"("append to file? (new file:F)"=TRUE, "2D data"=string[][] [["Note", "Duration"]] ("array")) -> ("new file path (Not A Path if cancelled)"=w712:path)  [unwired: 6 in]
        n316 = call-poly <vilib>:"Write To Spreadsheet File.vi"("append to file? (new file:F)"=TRUE, "2D data"=w713, "file path (dialog if empty)"=w712) -> ()  [unwired: 5 in, 1 out]
      }
    }
  }
  n317 = call "FYP_VI_MIDI_Close.vi"("midiOut"=w8) -> ()  [unwired: 6 in, 1 out]
